vi "JTAG Clock.vi"(1 "ACLK Divider":u16(ring) items=["/1"=0, "/2"=16, "/4"=32, "/8"=48], 2 "MCLK Divider":u16(ring) items=["/1"=0, "/2"=16, "/4"=32, "/8"=48], 3 "SMCLK Divider":u16(ring) items=["/1"=0, "/2"=2, "/4"=4, "/8"=6], 5 "ACLK Source":u16(ring) items=["LFXT1"=0, "VLOCLK"=32], 7 "MCLK Source":u16(ring) items=["DCOCLK"=0, "ACLK"=12], 9 "SMCLK Source":u16(ring) items=["DCOCLK"=0, "ACLK"=8], 11 "error in (no error)":errorcluster) -> (15 "error out":errorcluster)   [LabVIEW 2010]
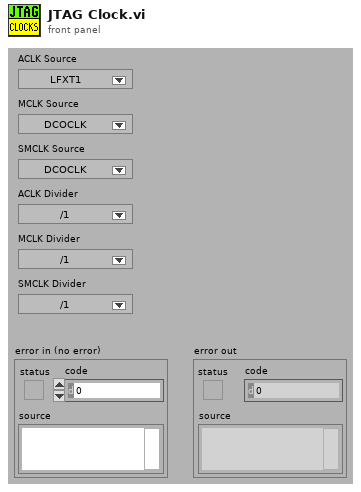
[diagram p1: front panel]
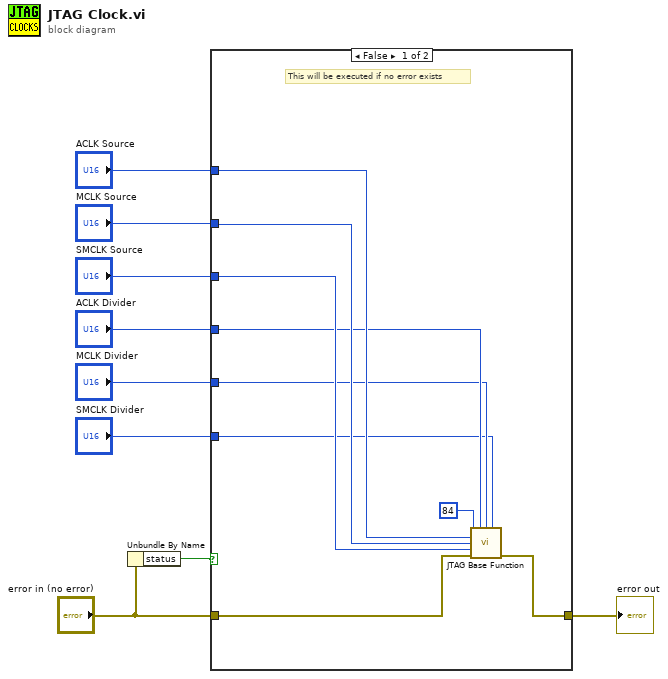
[diagram p0: block diagram]
diagram:
  n1 = Unbundle By Name("error in (no error)") -> ("status"=w8:bool)
  n2 = case shown="False" w8 {
    tunnel: [w17 w19] -> w9
    tunnel: "error in (no error)" -> [w18 w19]
    tunnel: "ACLK Source" -> [w16 _]
    tunnel: "MCLK Source" -> [w15 _]
    tunnel: "SMCLK Source" -> [w14 _]
    tunnel: "ACLK Divider" -> [w13 _]
    tunnel: "MCLK Divider" -> [w12 _]
    tunnel: "SMCLK Divider" -> [w11 _]
    frame False {
      # "This will be executed if no error exists"
      n3 = call "JTAG Base Function.vi"("Function"=84, "ARG 4"=w13, "ARG 5"=w12, "ARG 6"=w11, "ARG 1"=w16, "ARG 2"=w15, "ARG 3"=w14, "error in (no error)"=w18) -> ("error out"=w17:errorcluster)  [unwired: 5 in, 2 out]
    }
    frame True {
      # "Error exists, skip all functions"
    }
  }
  "error out" <- w9
